vi "Archive Target Data.vi"(8 "error in":errorcluster, 9 "Prefix":string, 10 "LBCB Number":T2, 11 "Data":T1) -> (0 "error out":errorcluster, 2 "string":string)   [LabVIEW 2009]
uses:
  Data Access Objects/Metadata/LBCB Number.ctl
  Mixed Mode Cartesian Data.ctl
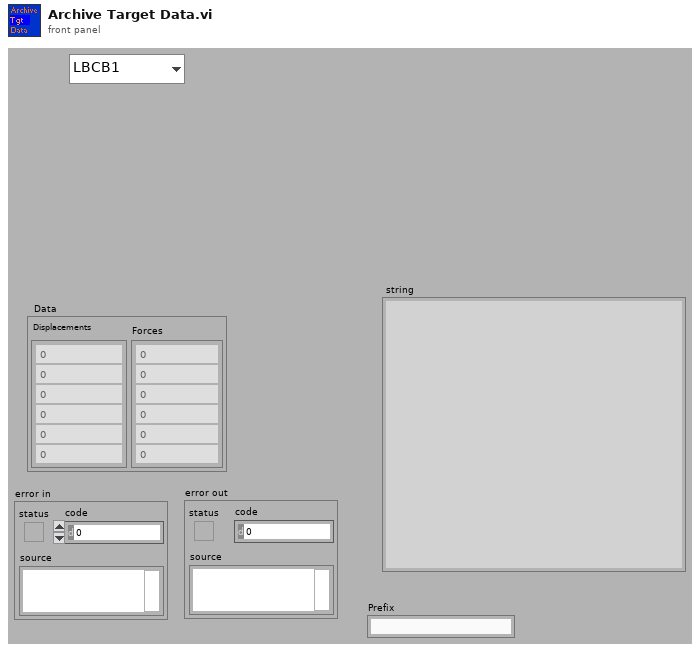
[diagram p1: front panel]
types:
  T1 = typedef "Mixed Mode Cartesian Data.ctl" = cluster{"Displacements":dbl[], "Forces":dbl[]}
  T2 = typedef "LBCB Number.ctl" = enum16{"LBCB1", "LBCB2"}
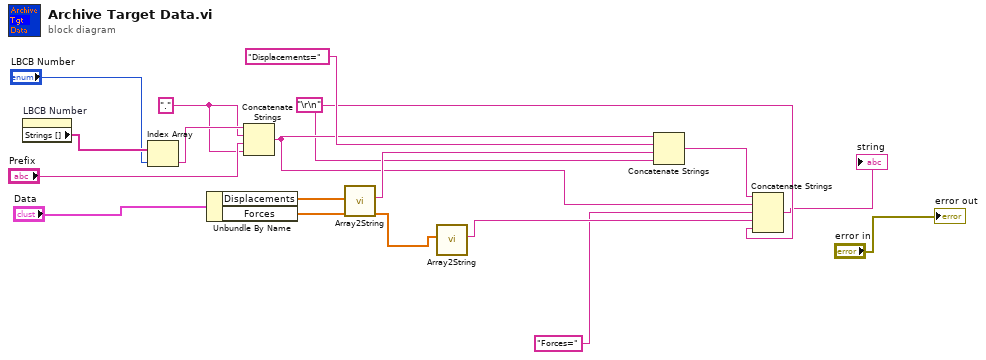
[diagram p0: block diagram]
diagram:
  w7 = "\r\n"
  w1 = "." ("string")
  n1 = property on="LBCB Number" class="Enum (strict)"() -> ("Strings []"=w17:string[])  [unwired: 2 in, 2 out]
  n2 = Index Array(array=w17, index="LBCB Number") -> (element=w5:string)
  n3 = Unbundle By Name("Data") -> ("Displacements"=w14:dbl[], "Forces"=w15:dbl[])
  n4 = Concatenate Strings(w5, w1, "Prefix", w1) -> (w11:string)
  n5 = call "Array2String.vi"("Array"=w14) -> ("String"=w12:string)  [unwired: 1 in, 9 out]
  n6 = call "Array2String.vi"("Array"=w15) -> ("String"=w10:string)  [unwired: 1 in, 9 out]
  n7 = Concatenate Strings(w11, "Displacements=", w12, w7) -> (w3:string)
  n8 = Concatenate Strings(w3, w11, "Forces=", w10, w7) -> (→"string":string)
  "error out" <- "error in"
